vi "Icon_Create Random Colors.vi"(8 "Error":errorcluster, 11 "Frame Select":enum32{"2 Color", "5 Color"}(ring)) -> (0 "Error Out":errorcluster, 3 "Color Out":T1)   [LabVIEW 2009]
doc: "Creates a random color cluster"
uses:
  Controls/Cluster/Cluster_Icon Color Set.ctl
  Controls/Enum/ENUM_Frame Template Select.ctl
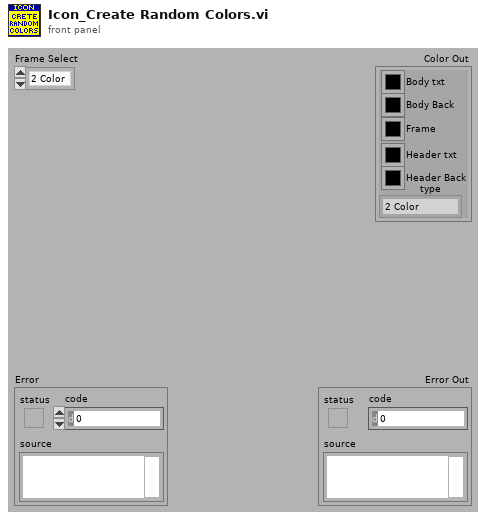
[diagram p1: front panel]
types:
  T1 = typedef "Cluster_Icon Color Set.ctl" = cluster{"Body txt":u32, "Body Back":u32, "Frame":u32, "Header txt":u32, "Header Back":u32, "type":T2}
  T2 = typedef "ENUM_Frame Template Select.ctl" = enum16{"2 Color", "5 Color"}
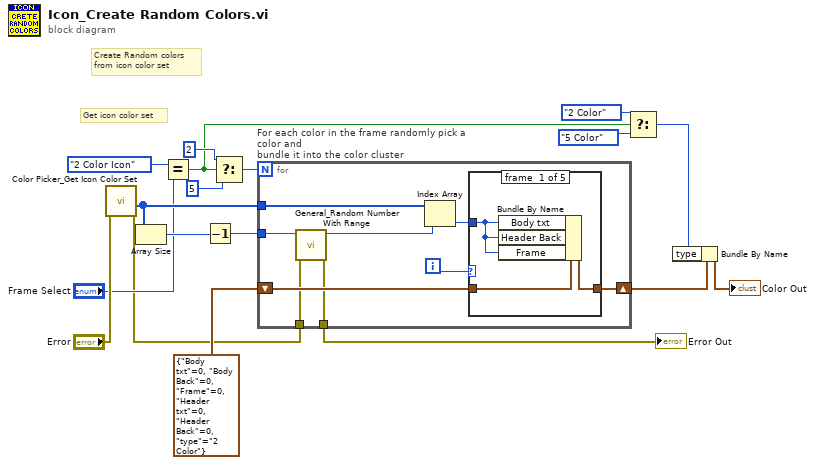
[diagram p0: block diagram]
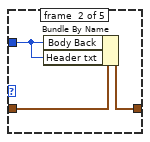
[diagram p2: hidden frame]
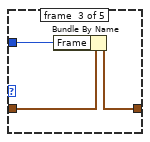
[diagram p3: hidden frame]
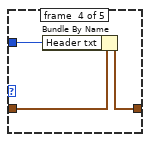
[diagram p4: hidden frame]
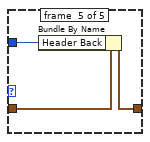
[diagram p5: hidden frame]
diagram:
  # "Get icon color set"
  # "Create Random colors\nfrom icon color set"
  n1 = call "Color Picker_Get Icon Color Set.vi"("Error"="Error") -> ("Error Out"=w2:errorcluster, "Icon Colors 1D Array Out"=w15:u32[])  [unwired: 8 in, 1 out]
  n2 = Array Size(array=w15) -> (size(s)=w17:i32)
  n3 = Equal?(x=enum32{"2 Color Icon", "5 Color Icon"}."2 Color Icon", y="Frame Select") -> (x = y?=w7:bool)
  n4 = Decrement(x=w17) -> (x-1=w16:i32)
  n5 = Select(t=2, s=w7, f=5) -> (s? t:f=w10:i32)
  n6 = for "For each color in the frame randomly pick a color and \nbundle it into the color cluster" {
    N: w10 -> [_]
    tunnel: w16 -> [w27]
    tunnel: w15 -> [w26]
    shift-right: [w23] -> w5
    shift-left: T1 {"Body txt"=0, "Body Back"=0, "Frame"=0, "Header txt"=0, "Header Back"=0, "type"=enum."2 Color"} ("Color") -> [w25]
    tunnel: w2 -> [w21]
    tunnel: [w20] -> w1
    i -> [w24]
    n7 = call "General_Random Number With Range.vi"("Error"=w21, "High (1.00)"=w27) -> ("Error Out"=w20:errorcluster, "Random # Out"=w19:i32)  [unwired: 8 in]
    n8 = Index Array(array=w26, index=w19) -> (element=w22:u32)
    n9 = case shown="1" w24 {
      tunnel: w25 -> [w30 w33 w36 w39 w42]
      tunnel: [w29 w32 w35 w38 w41] -> w23
      tunnel: w22 -> [w28 w31 w34 w37 w40]
      frame #0 {
        n10 = Bundle By Name(cluster=w30, "Body txt"=w28, "Header Back"=w28, "Frame"=w28) -> (w29:T1)
      }
      frame #1 {
        n11 = Bundle By Name(cluster=w33, "Body Back"=w31, "Header txt"=w31) -> (w32:T1)
      }
      frame #2 {
        n12 = Bundle By Name(cluster=w36, "Frame"=w34) -> (w35:T1)
      }
      frame #3 {
        n13 = Bundle By Name(cluster=w39, "Header txt"=w37) -> (w38:T1)
      }
      frame #4 {
        n14 = Bundle By Name(cluster=w42, "Header Back"=w40) -> (w41:T1)
      }
    }
  }
  "Error Out" <- w1
  n15 = Select(t=ENUM_Frame_Template_Select."2 Color" ("type"), s=w7, f=ENUM_Frame_Template_Select."5 Color") -> (s? t:f=w3:T2)
  n16 = Bundle By Name(cluster=w5, "type"=w3) -> (→"Color Out":T1)
